vi "Sign in tubes.vi"(8 "error in (no error)":errorcluster, 9 "Create By":string, 11 "connection information":path=path "D:/TUBES_SCADA_FIX/database.udl") -> (0 "error out":errorcluster, 2 "Cancel":bool)   [LabVIEW 2025]
uses:
  <vilib>/Alab Technologies/AES Crypto/Public VIs/String to Array.vi
  <vilib>/Alab Technologies/AES Crypto/Public VIs/Array to String.vi
  <vilib>/addons/database/Connection.llb/DB Tools Open Connec (Path).vi
  <vilib>/addons/database/Auxilliary.llb/DB Tools Format Datetime String (Time Stamp).vi
  <vilib>/addons/database/NI_Database_API.lvlib
  <vilib>/Alab Technologies/AES Crypto/AES Crypto.lvlib
panel:
  out "error out 2":errorcluster
  in  "error in (no error) 2":errorcluster
  in  "Tambahan":string
  out "Data tidak Kosong?":bool
  in  "Tab Control":enum32{"Page 1", "Page 2"}(tab)
  in  "Re Password":string
  in  "Cancel":bool
  in  "Ok Sign up":bool
  in  "Password":string
  in  "Username":string
  in  "Email":string
  in  "Nama":string
  in  "Role Supervisor":string(combo)
  in  "Role Engineer":string(combo)
  in  "stop":bool
  out "All data User":string
  out "Role data":string
  out "Hasil Query 2":string
  # "SELECT TOP (1000) [ID]\n      ,[Nama]\n      ,[Email]\n      ,[Nim]\n      ,[Username]\n      ,[Password]\n      ,[Role]\n  FROM [Praktikum_PIV].[dbo].[Table_Datauser]"
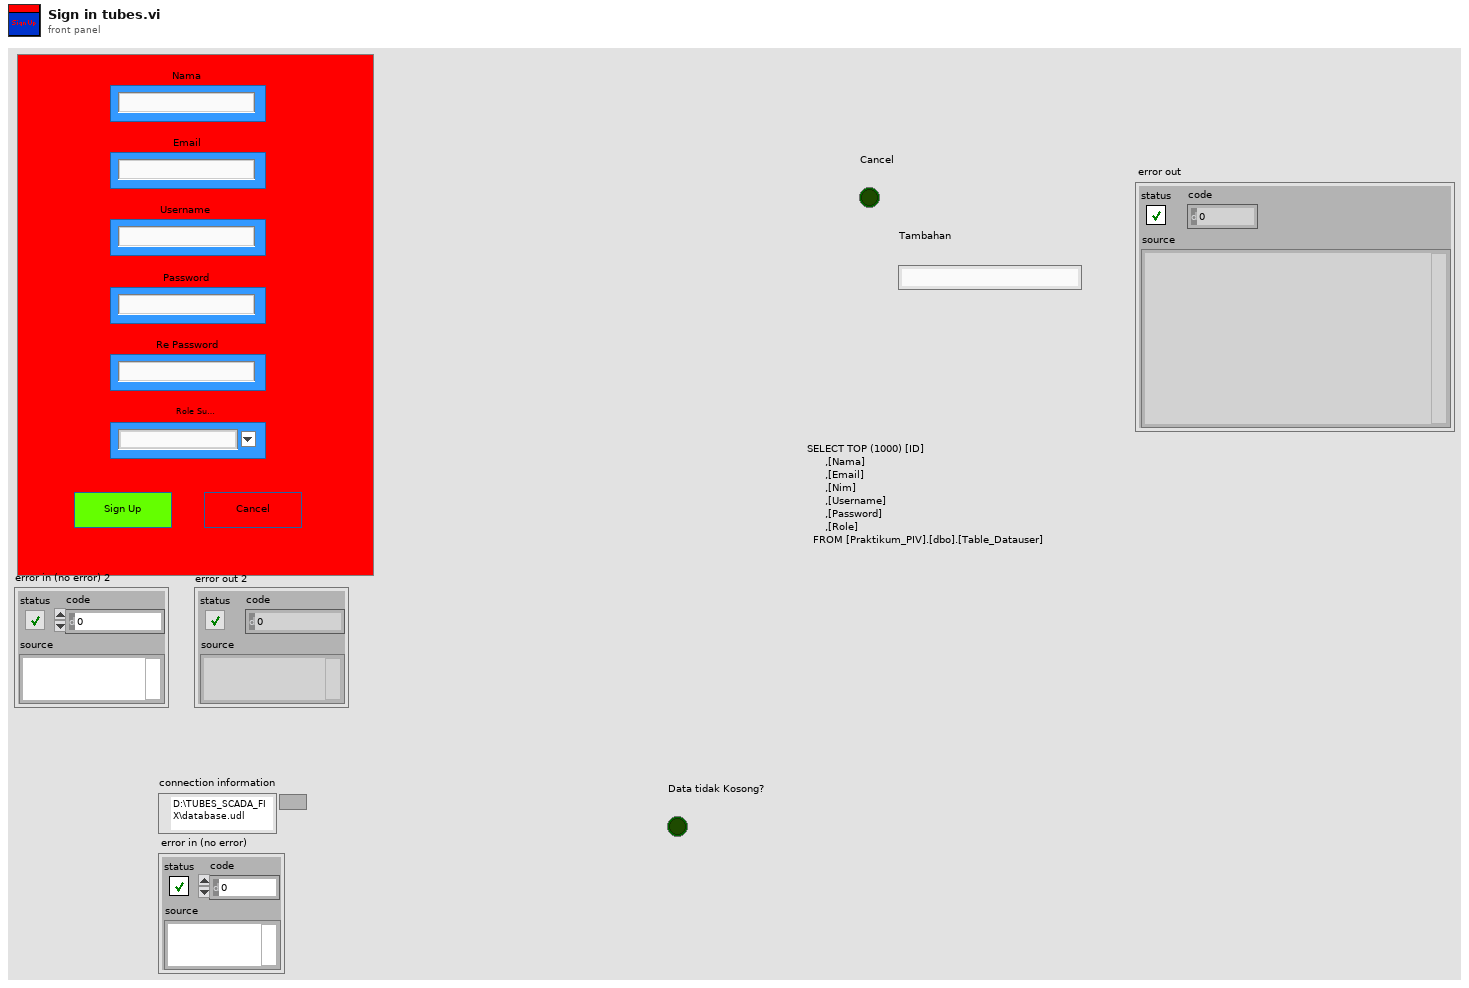
[diagram p1: front panel]
types:
  T1 = typedef "NI_Database_API.lvlib/Conn ObjectReference.ctl" = refnum<k1>
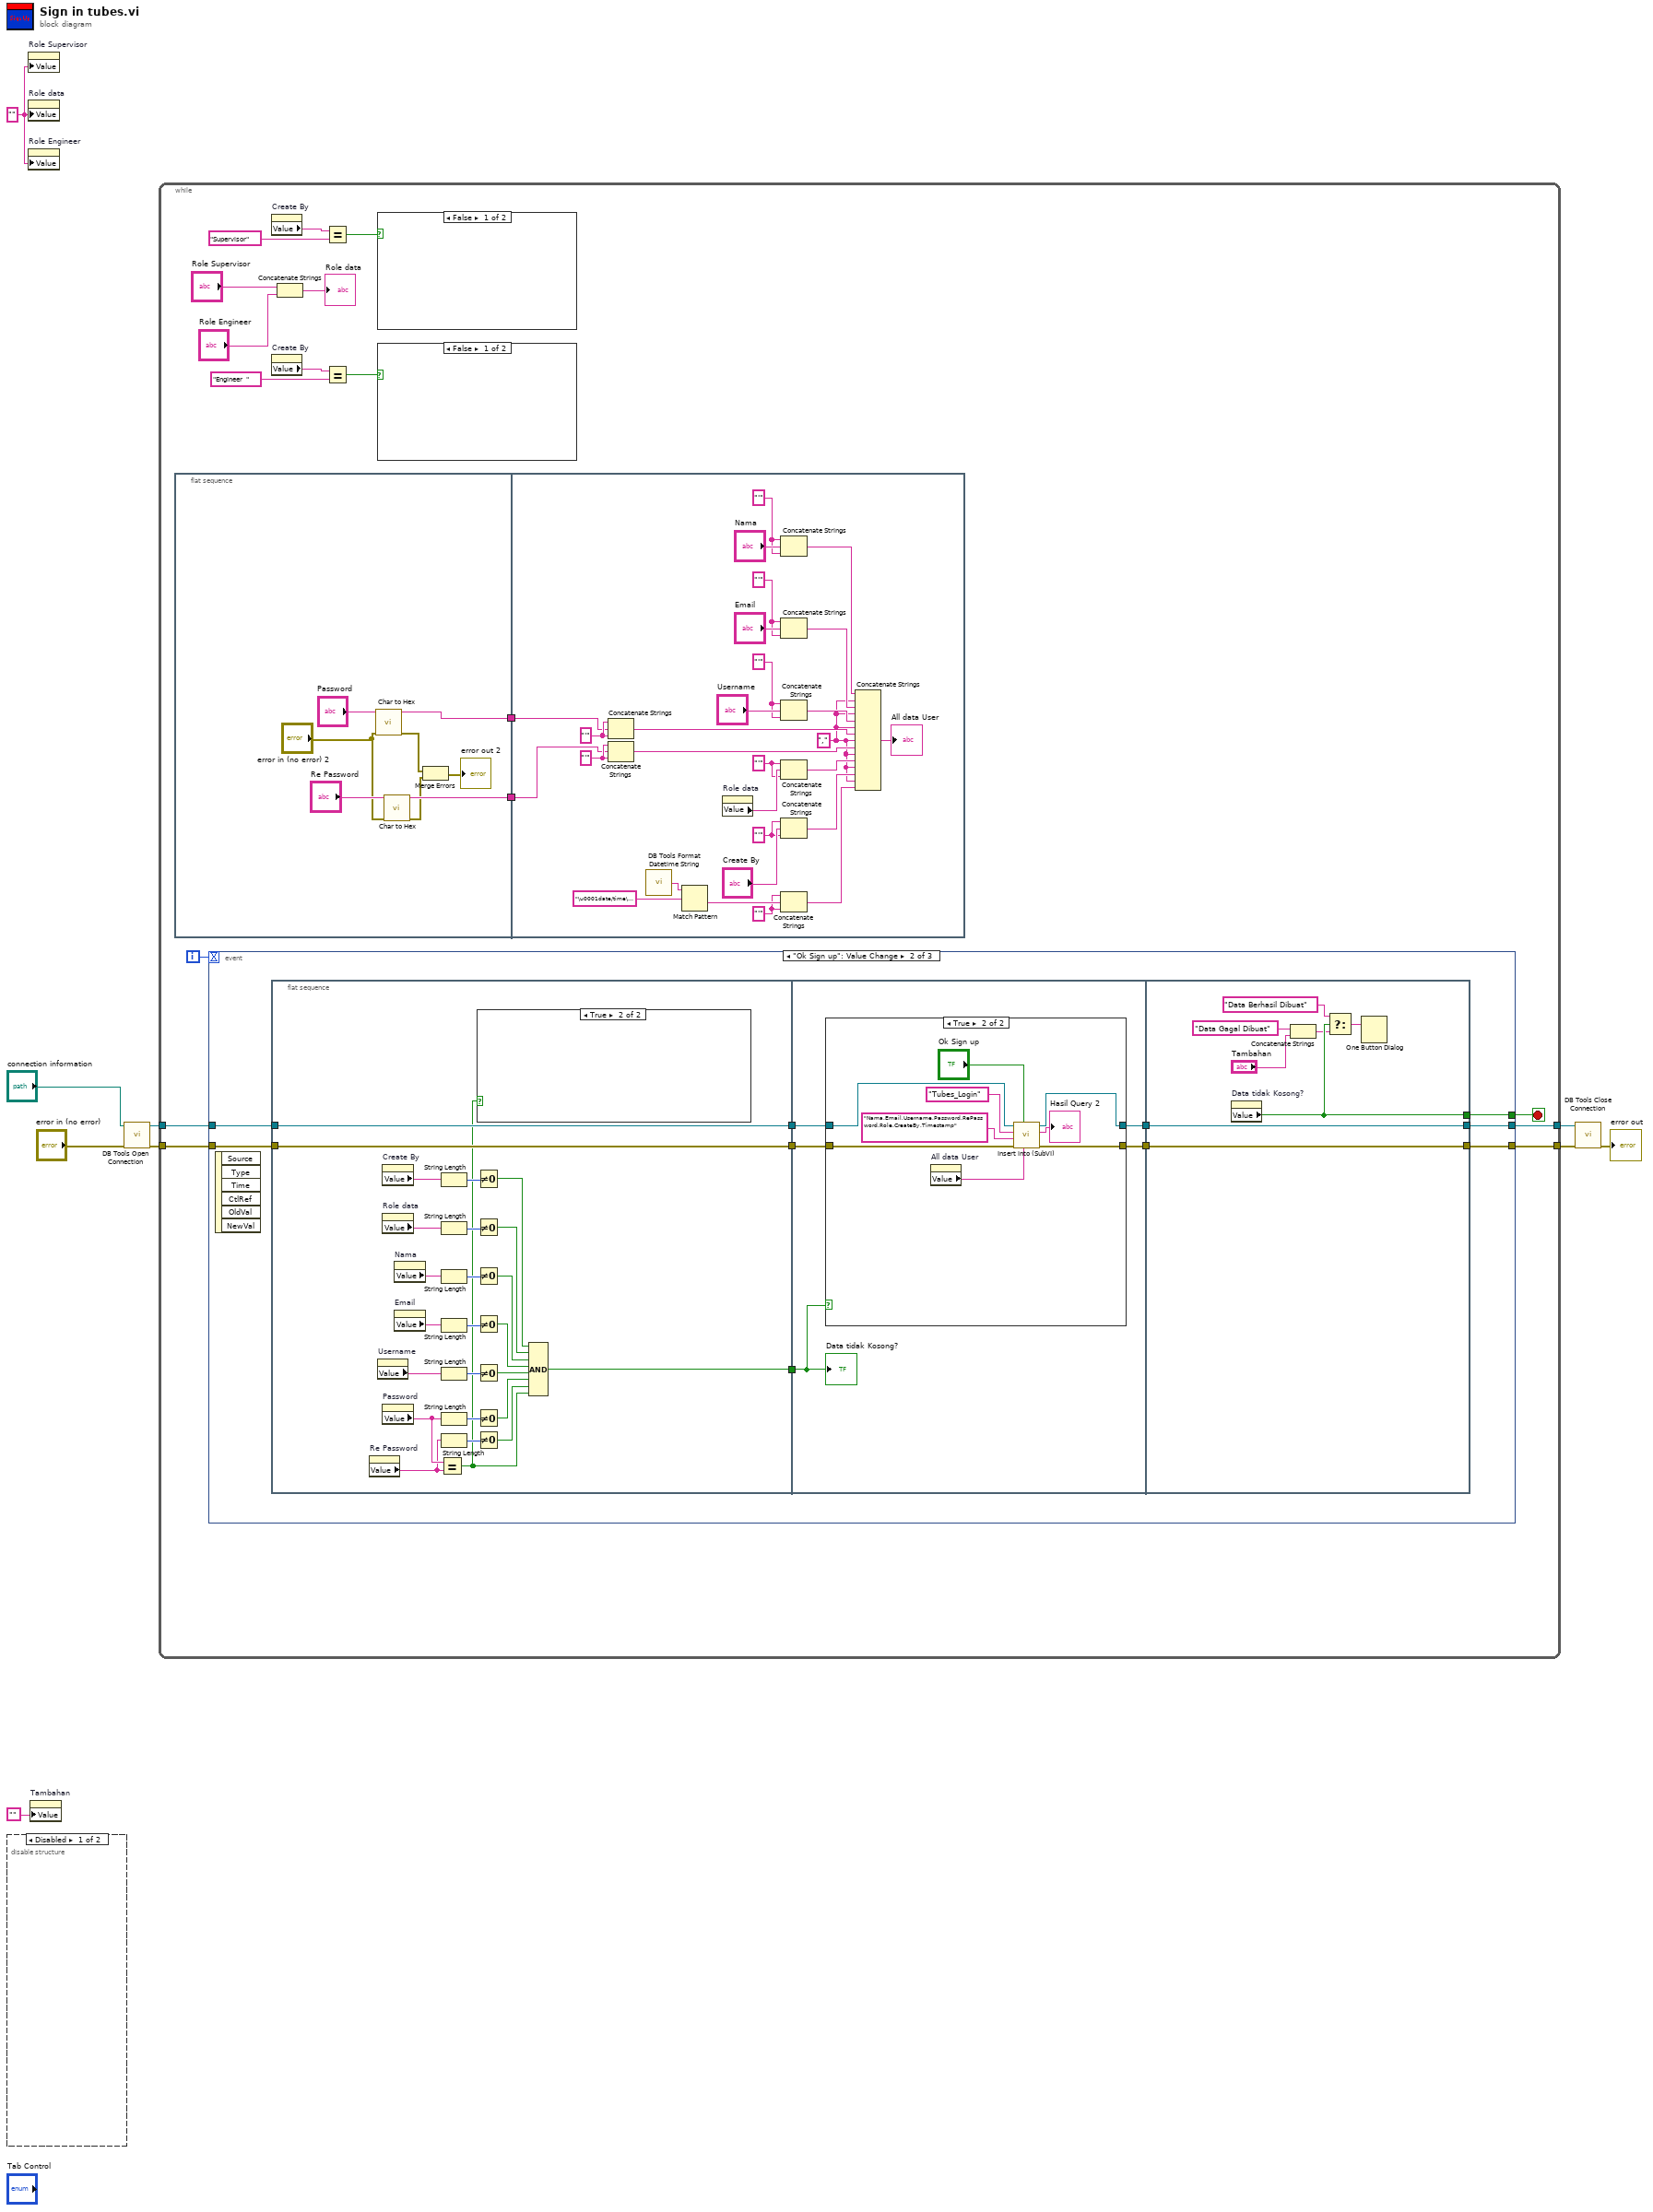
[diagram p0: block diagram]
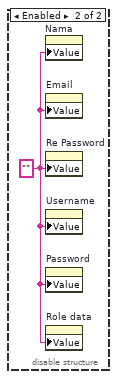
[diagram p2: hidden frame]
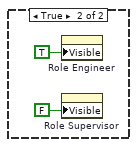
[diagram p3: hidden frame]
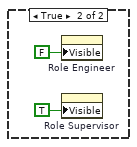
[diagram p4: hidden frame]
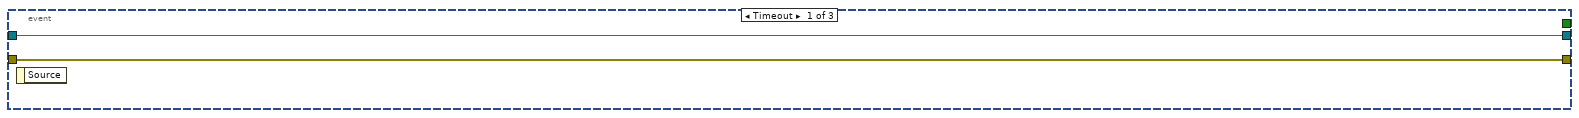
[diagram p5: hidden frame]
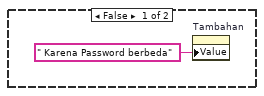
[diagram p6: hidden frame]
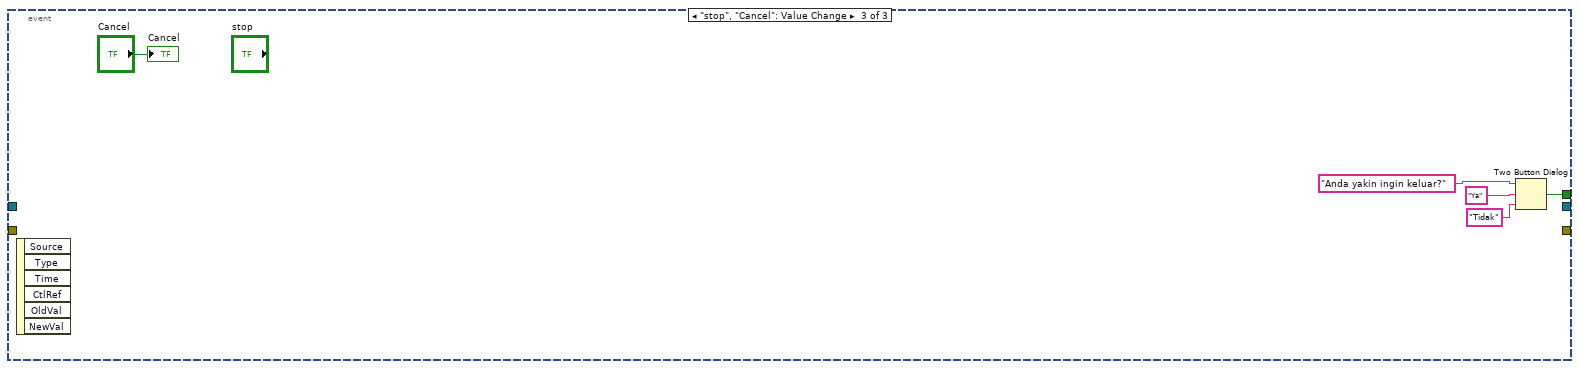
[diagram p8: hidden frame]
diagram:
  w2 = "" ("Role data")
  n1 = disable-structure shown="Disabled" {
    frame Disabled {
    }
    frame Enabled {
      w10 = ""
      n2 = property on="Nama" class="Str"("Value"=w10) -> ()  [unwired: 2 in, 2 out]
      n3 = property on="Email" class="Str"("Value"=w10) -> ()  [unwired: 2 in, 2 out]
      n4 = property on="Re Password" class="Str"("Value"=w10) -> ()  [unwired: 2 in, 2 out]
      n5 = property on="Username" class="Str"("Value"=w10) -> ()  [unwired: 2 in, 2 out]
      n6 = property on="Password" class="Str"("Value"=w10) -> ()  [unwired: 2 in, 2 out]
      n7 = property on="Role data" class="Str"("Value"=w10) -> ()  [unwired: 2 in, 2 out]
    }
  }
  n8 = property on="Role Supervisor" class="CmbBox"("Value"=w2) -> ()  [unwired: 2 in, 2 out]
  n9 = property on="Role data" class="Str"("Value"=w2) -> ()  [unwired: 2 in, 2 out]
  n10 = property on="Role Engineer" class="CmbBox"("Value"=w2) -> ()  [unwired: 2 in, 2 out]
  n11 = property on="Tambahan" class="Str"("Value"="") -> ()  [unwired: 2 in, 2 out]
  n12 = call-poly <vilib>:"DB Tools Open Connection.vi"("error in (no error)"="error in (no error)", "connection information"="connection information") -> ("error out"=w4:errorcluster, "connection reference"=w5:T1)  [unwired: 6 in]
  n13 = while {
    tunnel: w5 -> [w27]
    tunnel: [w26] -> w9
    tunnel: [w25] -> w8
    tunnel: w4 -> [w24]
    i -> [w22]
    stop <- w23 stop-if-true
    n14 = flat-sequence {
      tunnel: [w33] -> w12
      tunnel: [w32] -> w11
      tunnel: w12 -> [w40]
      tunnel: w11 -> [w44]
      frame #0 {
        n15 = call <vilib>:"Char to Hex.vi"("Input string (char)"="Password", "error in (no error)"="error in (no error) 2") -> ("Output string (hex)"=w33:string, "error out"=w30:errorcluster)  [unwired: 12 in]
        n16 = call <vilib>:"Char to Hex.vi"("Input string (char)"="Re Password", "error in (no error)"="error in (no error) 2") -> ("Output string (hex)"=w32:string, "error out"=w29:errorcluster)  [unwired: 12 in]
        n17 = Merge Errors(w30, w29) -> (→"error out 2":errorcluster)
      }
      frame #1 {
        w47 = "'" ("string")
        w45 = "'" ("string")
        w43 = "'" ("string")
        w42 = "'" ("string")
        w41 = "'" ("string")
        w39 = "'" ("string")
        w36 = "," ("string")
        w38 = "'" ("string")
        w37 = "'" ("string")
        n18 = Concatenate Strings(w41, w40, w41) -> (w53:string)
        n19 = Concatenate Strings(w45, w44, w45) -> (w58:string)
        n20 = call-poly <vilib>:"DB Tools Format Datetime String.vi"() -> ("date/time string"=w61:string)  [unwired: 1 in]
        n21 = Match Pattern(string=w61, regular expression="\u0001date/time\u0001") -> (after substring=w62:string)  [unwired: 1 in, 3 out]
        n22 = property on="Role data" class="Str"() -> ("Value"=w54:string)  [unwired: 2 in, 2 out]
        n23 = Concatenate Strings(w37, "Nama", w37) -> (w48:string)
        n24 = Concatenate Strings(w38, "Email", w38) -> (w50:string)
        n25 = Concatenate Strings(w39, "Username", w39) -> (w52:string)
        n26 = Concatenate Strings(w42, w54, w42) -> (w59:string)
        n27 = Concatenate Strings(w43, "Create By", w43) -> (w60:string)
        n28 = Concatenate Strings(w47, w62, w47) -> (w63:string)
        n29 = Concatenate Strings(w48, w36, w50, w36, w52, w36, w53, w36, w58, w36, w59, w36, w60, w36, w63) -> (→"All data User":string)
      }
    }
    n30 = event shown="[1] \"Ok Sign up\": Value Change" {
      selector: _ -> [_ _ _]
      dyn-events: _ -> [_ _ _]
      timeout: w22 -> [_ _ _]
      tunnel: w27 -> [w69 w79 _]
      tunnel: [w69 w78 _] -> w26
      tunnel: [w68 w76 _] -> w25
      tunnel: w24 -> [w68 w77 _]
      tunnel: [_ w70 w131] -> w23
      event Timeout {
        n31 = event-data() -> ()  [unwired: 1 in, 1 out]
      }
      event "Ok Sign up": Value Change {
        n32 = event-data() -> ()  [unwired: 1 in, 6 out]
        n33 = flat-sequence {
          tunnel: w77 -> [w103]
          tunnel: w79 -> [w104]
          tunnel: [w104] -> w73
          tunnel: [w103] -> w72
          tunnel: [w89] -> w71
          tunnel: [w109] -> w75
          tunnel: [w107] -> w74
          tunnel: w73 -> [w110]
          tunnel: w72 -> [w108]
          tunnel: w71 -> [w106]
          tunnel: [w128] -> w76
          tunnel: [w129] -> w78
          tunnel: w75 -> [w129]
          tunnel: w74 -> [w128]
          tunnel: [w125] -> w70
          frame #0 {
            n34 = property on="Re Password" class="Str"() -> ("Value"=w85:string)  [unwired: 2 in, 2 out]
            n35 = property on="Username" class="Str"() -> ("Value"=w97:string)  [unwired: 2 in, 2 out]
            n36 = property on="Create By" class="Str"() -> ("Value"=w92:string)  [unwired: 2 in, 2 out]
            n37 = property on="Role data" class="Str"() -> ("Value"=w94:string)  [unwired: 2 in, 2 out]
            n38 = property on="Password" class="Str"() -> ("Value"=w86:string)  [unwired: 2 in, 2 out]
            n39 = property on="Nama" class="Str"() -> ("Value"=w101:string)  [unwired: 2 in, 2 out]
            n40 = property on="Email" class="Str"() -> ("Value"=w99:string)  [unwired: 2 in, 2 out]
            n41 = Equal?(x=w86, y=w85) -> (x = y?=w84:bool)
            n42 = String Length(string=w92) -> (length=w93:i32)
            n43 = String Length(string=w94) -> (length=w95:i32)
            n44 = String Length(string=w101) -> (length=w102:i32)
            n45 = String Length(string=w99) -> (length=w100:i32)
            n46 = String Length(string=w97) -> (length=w98:i32)
            n47 = String Length(string=w86) -> (length=w96:i32)
            n48 = String Length(string=w85) -> (length=w88:i32)
            n49 = Not Equal To 0?(x=w93) -> (x != 0?=w80:bool)
            n50 = Not Equal To 0?(x=w95) -> (x != 0?=w81:bool)
            n51 = Not Equal To 0?(x=w102) -> (x != 0?=w82:bool)
            n52 = Not Equal To 0?(x=w100) -> (x != 0?=w83:bool)
            n53 = Not Equal To 0?(x=w98) -> (x != 0?=w91:bool)
            n54 = Not Equal To 0?(x=w96) -> (x != 0?=w90:bool)
            n55 = Not Equal To 0?(x=w88) -> (x != 0?=w87:bool)
            n56 = case shown="True" w84 {
              frame False {
                n57 = property on="Tambahan" class="Str"("Value"=" Karena Password berbeda" ("Tambahan")) -> ()  [unwired: 2 in, 2 out]
              }
              frame True {
              }
            }
            n58 = Compound Arithmetic op=AND(w80, w81, w82, w83, w91, w90, w87, w84) -> (w89:bool)
          }
          frame #1 {
            n59 = case shown="True" w106 {
              tunnel: w110 -> [w112 w121]
              tunnel: [w112 w120] -> w109
              tunnel: w108 -> [w111 w119]
              tunnel: [w111 w117] -> w107
              frame False {
              }
              frame True {
                n60 = property on="All data User" class="Str"() -> ("Value"=w116:string)  [unwired: 2 in, 2 out]
                n61 = call "Insert into (SubVI).vi"("Nilai Data"=w116, "Kirim Data?"="Ok Sign up", "error in (no error)"=w119, "Coumn"="Nama,Email,Username,Password,RePassword,Role,CreateBy,Timestamp", "Nama Table"="Tubes_Login", "Refnum in"=w121) -> ("error out"=w117:errorcluster, "Hasil Query"=→"Hasil Query 2":string, "Refnum out"=w120:T1)  [unwired: 3 in]
              }
            }
            "Data tidak Kosong?" <- w106
          }
          frame #2 {
            n62 = property on="Data tidak Kosong?" class="Bool (strict)"() -> ("Value"=w125:bool)  [unwired: 2 in, 2 out]
            n63 = Concatenate Strings("Data Gagal Dibuat", "Tambahan") -> (w124:string)
            n64 = Select(t="Data Berhasil Dibuat", s=w125, f=w124) -> (s? t:f=w126:string)
            n65 = One Button Dialog(message=w126) -> ()  [unwired: 1 in, 1 out]
          }
        }
      }
      event "stop", "Cancel": Value Change {
        n66 = event-data() -> ()  [unwired: 1 in, 6 out]
        n67 = Two Button Dialog(message="Anda yakin ingin keluar?", 1:"Tidak" ("F button name (\"Cancel\")"), 2:"Ya" ("T button name (\"OK\")")) -> (T button?=w131:bool)
        "Cancel" <- "Cancel"
      }
    }
    n68 = property on="Create By" class="Str"() -> ("Value"=w18:string)  [unwired: 2 in, 2 out]
    n69 = property on="Create By" class="Str"() -> ("Value"=w16:string)  [unwired: 2 in, 2 out]
    n70 = Concatenate Strings("Role Supervisor", "Role Engineer") -> (→"Role data":string)
    n71 = Equal?(x=w18, y="Supervisor") -> (x = y?=w17:bool)
    n72 = Equal?(x=w16, y="Engineer  ") -> (x = y?=w15:bool)
    n73 = case shown="False" w17 {
      frame False {
      }
      frame True {
        n74 = property on="Role Engineer" class="CmbBox"("Visible"=FALSE) -> ()  [unwired: 2 in, 2 out]
        n75 = property on="Role Supervisor" class="CmbBox"("Visible"=TRUE) -> ()  [unwired: 2 in, 2 out]
      }
    }
    n76 = case shown="False" w15 {
      frame False {
      }
      frame True {
        n77 = property on="Role Engineer" class="CmbBox"("Visible"=TRUE) -> ()  [unwired: 2 in, 2 out]
        n78 = property on="Role Supervisor" class="CmbBox"("Visible"=FALSE) -> ()  [unwired: 2 in, 2 out]
      }
    }
  }
  n79 = call <vilib>:"DB Tools Close Connection.vi"("error in (no error)"=w8, "connection reference"=w9) -> ("error out"=→"error out":errorcluster)  [unwired: 5 in]
